vi "AxisNo2PhysName.vi"(8 "error in (no error)":errorcluster, 10 "AxisNumber":u8, 11 "CS++Motor in":refnum<class "CS++Motor.lvclass">) -> (0 "error out":errorcluster, 2 "PhysicalChannelName":string, 3 "CS++Motor out":refnum<class "CS++Motor.lvclass">)   [LabVIEW 2016, in "CS++Motor.lvlib" / "CS++Motor.lvclass"]
doc: "This small utility VI needs the axis number (0...N-1) and returns the physical Name of the channel. This is probably needed in all child classes of CS++Motor.lvclass."
uses:
  CS++Motor.lvclass
  CS++Motor.lvclass/CS++Motor.ctl
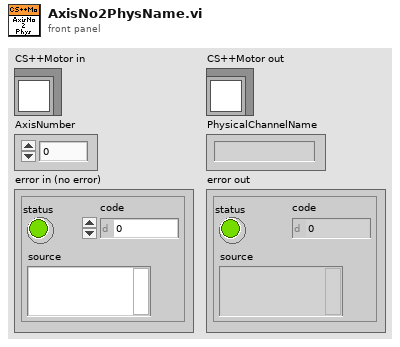
[diagram p1: front panel]
types:
  T1 = cluster{"LogicalName":string, "PhysicalName":string, "unit":string, "Scaling":dbl, "Scaling Offset":dbl, "StartVelocity":dbl, "StopVelocity":dbl, "Acceleration":dbl, "RangeMin":dbl, "RangeMax":dbl, "LogicalPos-Array":cluster{"LogicalPosition":string, "SetPosition":dbl}[]}[]
  T2 = cluster{"LogicalName":string, "PhysicalName":string, "unit":string, "Scaling":dbl, "Scaling Offset":dbl, "StartVelocity":dbl, "StopVelocity":dbl, "Acceleration":dbl, "RangeMin":dbl, "RangeMax":dbl, "LogicalPos-Array":cluster{"LogicalPosition":string, "SetPosition":dbl}[]}
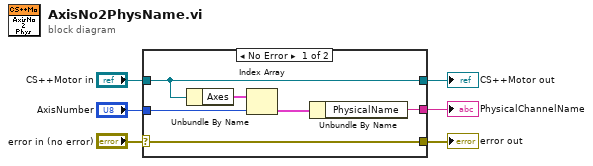
[diagram p0: block diagram]
diagram:
  n1 = case shown="No Error" "error in (no error)" {
    selector: "error in (no error)" -> [w12 w14]
    tunnel: [w12 w14] -> w5
    tunnel: [w11 w13] -> w3
    tunnel: "CS++Motor in" -> [w11 w13]
    tunnel: "AxisNumber" -> [w9 _]
    tunnel: [w7 _] -> w1
    frame No Error {
      n2 = Unbundle By Name(w11) -> ("Axes"=w10:T1)
      n3 = Index Array(array=w10, index=w9) -> (element=w8:T2)
      n4 = Unbundle By Name(w8) -> ("PhysicalName"=w7:string)
    }
    frame Error {
    }
  }
  "error out" <- w5
  "CS++Motor out" <- w3
  "PhysicalChannelName" <- w1
